vi "timeSeries.vi"(0 "Results Path":string="C:\\Users\\Hesham\\Desktop\\Analyse WT Data\\C1\\tmseries\\node1\\") -> (1 "Mean VRs":dbl[][](array[numeric]), 2 "GEM VRs":dbl[][](array[numeric]))   [LabVIEW 2018]
uses:
  <vilib>/Analysis/3filter.llb/Filter Passband Type.ctl
  <vilib>/Analysis/baseanly.llb/Mean (DBL).vi
  <vilib>/Utility/file.llb/Read Delimited Spreadsheet (string).vi
  <vilib>/Analysis/3filter.llb/Butterworth Filter (DBL).vi
  <vilib>/Analysis/NI_AALBase.lvlib
panel:
  out "Iteration":i32
  out "Input VR RMS":dbl[][](array[numeric])
  out "Input VR AVG":dbl[][](array[numeric])
  out "Processed Array - RMS":dbl[][](array[numeric])
  out "Processed Array - Means":dbl[][](array[numeric])
  out "Raw Array":sgl[][][](array[numeric])
  out "path":path
  out "Data":sgl[](graph)
  # "TO DO:\n- Add MF and AF to the probability calculation\n- Probes that have moved/removed"
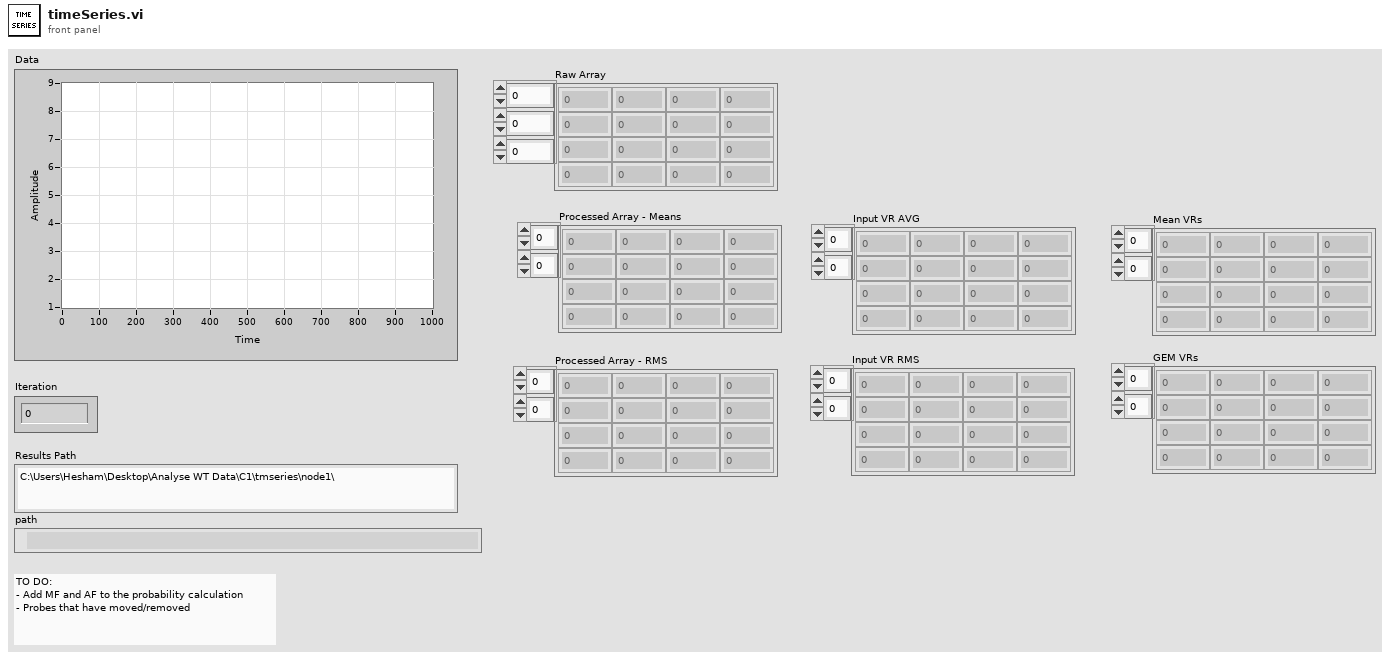
[diagram p1: front panel]
types:
  T1 = enum16{"big-endian, network order", "native, host order", "little-endian"}
  T2 = typedef "NI_AALBase.lvlib/Filter Passband Type.ctl" = enum32{"Lowpass", "Highpass", "Bandpass", "Bandstop"}
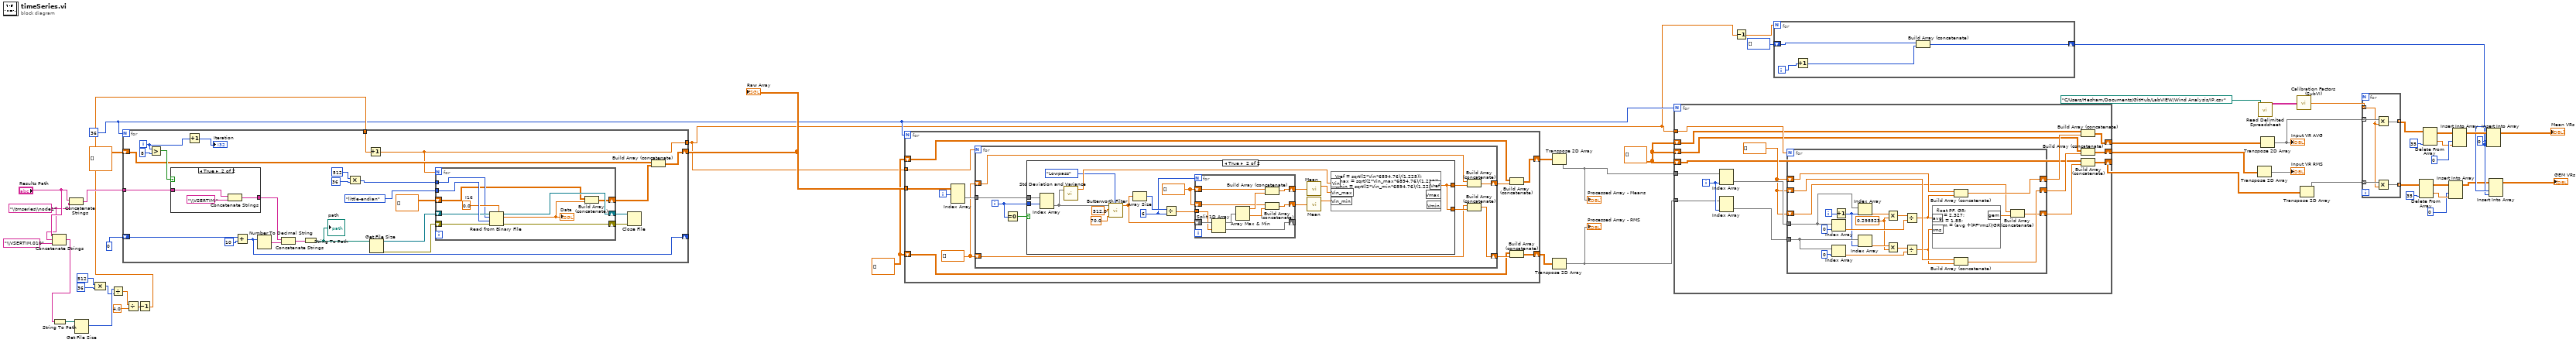
[diagram p0: block diagram]
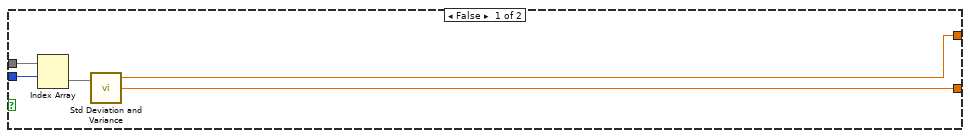
[diagram p2: hidden frame]
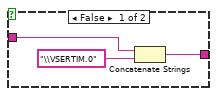
[diagram p3: hidden frame]
diagram:
  w4 = 0 ("disabled index (col)")
  w10 = 36
  w22 = "\\tmseries\\node1"
  w37 = dbl[][] []
  w42 = dbl[][] []
  n1 = Concatenate Strings("Results Path", w22, "\\VSERTIM.010" ("string")) -> (w20:string)
  n2 = String To Path(string=w20) -> (path=w19:path)
  n3 = Concatenate Strings("Results Path", w22) -> (w24:string)
  n4 = Get File Size(file=w19) -> (size (in bytes)=w18:i64)  [unwired: 1 in, 2 out]
  n5 = Compound Arithmetic op=MULTIPLY(512, 36 ("y")) -> (w15:i32)
  n6 = Divide(x=w18, y=w15) -> (x/y=w14:dbl)
  n7 = Divide(x=w14, y=4.0) -> (x/y=w12:dbl)
  n8 = Decrement(x=w12) -> (x-1=w11:dbl)
  n9 = for {
    N: w10 -> [_]
    shift-right: [w67] -> _
    shift-left: 0 -> [w68]
    tunnel: w24 -> [w64]
    shift-right: [w60] -> w50
    shift-left: sgl[][][] [] -> [w59]
    tunnel: [w57] -> w9
    tunnel: w11 -> [w53]
    i -> [w56]
    n10 = Greater?(x=w56, y=8) -> (0:w71:bool)
    n11 = case shown="True" w71 {
      tunnel: [w79 w82] -> w62
      tunnel: w64 -> [w81 w84]
      frame False {
        n12 = Concatenate Strings(w81, "\\VSERTIM.0") -> (w79:string)
      }
      frame True {
        n13 = Concatenate Strings(w84, "\\VSERTIM." ("string")) -> (w82:string)
      }
    }
    n14 = Increment(x=w56) -> (x+1=→"Iteration":i32)
    n15 = Add(x=w68, y=10) -> (x+y=w67:i32)
    n16 = Number To Decimal String(number=w67) -> (decimal integer string=w63:string)  [unwired: 1 in]
    n17 = Concatenate Strings(w62, w63) -> (w66:string)
    n18 = String To Path(string=w66) -> (path=w65:path)
    "path" <- w65
    n19 = Compound Arithmetic op=MULTIPLY(512, 36 ("y")) -> (w54:i32)
    n20 = Increment(x=w53) -> (x+1=w57:dbl)
    n21 = Get File Size(file=w65) -> (refnum out=w76:refnum<file>, 0:w77:errorcluster)  [unwired: 1 in, 1 out]
    n22 = for {
      N: w57 -> [_]
      tunnel: T1."little-endian" ("Byte Order") -> [w94]
      shift-right: [w89] -> w74
      shift-left: w77 -> [w93]
      shift-right: [w90] -> w75
      shift-left: w76 -> [w92]
      tunnel: w54 -> [w88]
      shift-right: [w86] -> w58
      shift-left: sgl[][] [] -> [w85]
      w91 = sgl 0.0  # I16
      n23 = Read from Binary File(5:w91, 8:w93, 9:w94, 10:w88, 11:w92) -> (0:w89:errorcluster, 2:w87:sgl[], 3:w90:refnum<file>)  [unwired: 1 in, 1 out]
      "Data" <- w87
      n24 = Build Array (concatenate)(w85, w87) -> (w86:sgl[][])
    }
    n25 = Close File(refnum=w75, error in=w74) -> ()  [unwired: 2 out]
    n26 = Build Array (concatenate)(w59, w58) -> (w60:sgl[][][])
  }
  "Raw Array" <- w50
  n27 = for {
    N: w10 -> [_]
    tunnel: w50 -> [w105]
    tunnel: w9 -> [w103]
    shift-right: [w101] -> w49
    shift-left: w42 -> [w100]
    shift-right: [w98] -> w48
    shift-left: w42 -> [w97]
    i -> [w104]
    w95 = dbl[] []
    n28 = Index Array(array=w105, index (dim 0)=w104) -> (element=w96:sgl[][])  [unwired: 2 in]
    n29 = for {
      N: w103 -> [_]
      tunnel: w96 -> [w111]
      shift-right: [w114] -> w102
      shift-left: w95 -> [w107]
      shift-right: [w113] -> w99
      shift-left: w95 -> [w106]
      i -> [w110]
      n30 = Equal To 0?(x=w110) -> (x = 0?=w112:bool)
      n31 = case shown="True" w112 {
        tunnel: w110 -> [w116 w136]
        tunnel: w111 -> [w119 w135]
        tunnel: [w117 w124] -> w108
        tunnel: [w118 w124] -> w109
        frame False {
          n32 = Index Array(array=w119, index (row)=w116) -> (element=w115:sgl[])  [unwired: 1 in]
          n33 = call <vilib>:"Std Deviation and Variance.vi"("X"=w115) -> ("mean"=w117:dbl, "standard deviation"=w118:dbl)  [unwired: 1 in, 1 out]
        }
        frame True {
          w127 = dbl[] []
          w122 = 6
          n34 = Index Array(array=w135, index (row)=w136) -> (element=w128:sgl[])  [unwired: 1 in]
          n35 = call <vilib>:"Std Deviation and Variance.vi"("X"=w128) -> ("mean"=w134:dbl)  [unwired: 1 in, 2 out]
          n36 = call-poly <vilib>:"Butterworth Filter.vi"("filter type"=Filter_Passband_Type."Lowpass", "low cutoff freq: fl"=70.0, "sampling freq: fs"=512.0, "X"=w128) -> ("Filtered X"=w121:dbl[])  [unwired: 4 in, 1 out]
          n37 = Array Size(array=w121) -> (size(s)=w123:i32)
          n38 = Divide(x=w123, y=w122) -> (x/y=w120:dbl)
          n39 = for {
            N: w122 -> [_]
            shift-right: [w145] -> _
            shift-left: w121 -> [w146]
            shift-right: [w144] -> w130
            shift-left: w127 -> [w141]
            shift-right: [w142] -> w129
            shift-left: w127 -> [w138]
            tunnel: w120 -> [w137]
            n40 = Split 1D Array(array=w146, index=w137) -> (first subarray=w143:dbl[], second subarray=w145:dbl[])
            n41 = Array Max & Min(array=w143) -> (max value=w140:dbl, min value=w139:dbl)  [unwired: 2 out]
            n42 = Build Array (concatenate)(w141, w140) -> (w144:dbl[])
            n43 = Build Array (concatenate)(w138, w139) -> (w142:dbl[])
          }
          n44 = call-poly <vilib>:"Mean.vi"("X"=w130) -> ("mean"=w126:dbl)  [unwired: 1 out]
          n45 = call-poly <vilib>:"Mean.vi"("X"=w129) -> ("mean"=w125:dbl)  [unwired: 1 out]
          n46 = formula code="Vref = sqrt((2*Vin*6894.76)/(1.225));\nVmax = sqrt((2*Vin_max*6894.76)/(1.225));\nVmin = sqrt((2*Vin_min*6894.76)/(1.225));"("Vin"=w134, "Vin_max"=w126, "Vin_min"=w125) -> ("Vref"=w124:dbl)  [unwired: 2 out]
        }
      }
      n47 = Build Array (concatenate)(w107, w108) -> (w114:dbl[])
      n48 = Build Array (concatenate)(w106, w109) -> (w113:dbl[])
    }
    n49 = Build Array (concatenate)(w100, w102) -> (w101:dbl[][])
    n50 = Build Array (concatenate)(w97, w99) -> (w98:dbl[][])
  }
  n51 = Transpose 2D Array(2D array=w49) -> (transposed array=w47:dbl[][])
  "Processed Array - Means" <- w47
  n52 = Transpose 2D Array(2D array=w48) -> (transposed array=w43:dbl[][])
  "Processed Array - RMS" <- w43
  n53 = for {
    N: w10 -> [_]
    tunnel: w47 -> [w157]
    tunnel: w9 -> [w161]
    shift-right: [w155] -> w46
    shift-left: w37 -> [w159]
    shift-right: [w153] -> w45
    shift-left: w37 -> [w152]
    tunnel: w43 -> [w151]
    shift-right: [w148] -> w36
    shift-left: w37 -> [w147]
    i -> [w158]
    w150 = dbl[] []
    n54 = Index Array(array=w157, index (col)=w158) -> (element=w162:dbl[])  [unwired: 1 in]
    n55 = Index Array(array=w151, index (col)=w158) -> (element=w156:dbl[])  [unwired: 1 in]
    n56 = for {
      N: w161 -> [_]
      tunnel: w162 -> [w176]
      shift-right: [w181] -> w160
      shift-left: w150 -> [w180]
      tunnel: w156 -> [w175]
      shift-right: [w170] -> w154
      shift-left: w150 -> [w169]
      shift-right: [w164] -> w149
      shift-left: w150 -> [w163]
      i -> [w183]
      w168 = 0.298523 ("y")
      n57 = Index Array(array=w176, index=0 ("index (row)")) -> (element=w182:dbl)
      n58 = Index Array(array=w175, index=0 ("index (row)")) -> (element=w172:dbl)
      n59 = Increment(x=w183) -> (x+1=w174:i32)
      n60 = Index Array(array=w176, index=w174) -> (element=w179:dbl)
      n61 = Index Array(array=w175, index=w174) -> (element=w171:dbl)
      n62 = Multiply(x=w179, y=w168) -> (x*y=w178:dbl)
      n63 = Multiply(x=w171, y=w168) -> (x*y=w173:dbl)
      n64 = Divide(x=w178, y=w182) -> (x/y=w167:dbl)
      n65 = Divide(x=w173, y=w172) -> (x/y=w166:dbl)
      n66 = formula code="float PF, GR; \nPF = 2.327;\nGR = 1.85;\ngem = (avg +(PF*rms))/GR;"("avg"=w167, "rms"=w166) -> ("gem"=w165:dbl)
      n67 = Build Array (concatenate)(w180, w167) -> (w181:dbl[])
      n68 = Build Array (concatenate)(w169, w166) -> (w170:dbl[])
      n69 = Build Array (concatenate)(w163, w165) -> (w164:dbl[])
    }
    n70 = Build Array (concatenate)(w159, w160) -> (w155:dbl[][])
    n71 = Build Array (concatenate)(w152, w154) -> (w153:dbl[][])
    n72 = Build Array (concatenate)(w147, w149) -> (w148:dbl[][])
  }
  n73 = Decrement(x=w9) -> (x-1=w8:dbl)
  n74 = for {
    N: w8 -> [_]
    shift-right: [w188] -> w3
    shift-left: i32[] [] -> [w187]
    i -> [w186]
    n75 = Increment(x=w186) -> (x+1=w185:i32)
    n76 = Build Array (concatenate)(w187, w185) -> (w188:i32[])
  }
  n77 = Transpose 2D Array(2D array=w45) -> (transposed array=→"Input VR RMS":dbl[][])
  n78 = call-poly <vilib>:"Read Delimited Spreadsheet.vi"("file path (dialog if empty)"=path "C:/Users/Hesham/Documents/GitHub/LabVIEW/Wind Analysis/IP.csv") -> ("all rows"=w41:string[][])  [unwired: 9 in, 5 out]
  n79 = Transpose 2D Array(2D array=w46) -> (transposed array=w39:dbl[][])
  "Input VR AVG" <- w39
  n80 = call "Calibration Factors (SubVI).vi"("IP List"=w41) -> ("Calibration Factors"=w38:dbl[])
  n81 = Transpose 2D Array(2D array=w36) -> (transposed array=w35:dbl[][])
  n82 = for {
    tunnel: w39 -> [w193] mode=indexing
    tunnel: w38 -> [w190] mode=indexing
    tunnel: [w192] -> w33 mode=indexing
    tunnel: w35 -> [w191] mode=indexing
    tunnel: [w189] -> w25 mode=indexing
    n83 = Multiply(x=w193, y=w190) -> (x*y=w192:dbl[])
    n84 = Multiply(x=w191, y=w190) -> (x*y=w189:dbl[])
  }
  n85 = Delete From Array(array=w25, index (col)=35 ("disabled index (col)")) -> (deleted portion=w29:dbl[], array with subset deleted=w27:dbl[][])  [unwired: 2 in]
  n86 = Delete From Array(array=w33, index (col)=35 ("disabled index (col)")) -> (deleted portion=w30:dbl[], array with subset deleted=w32:dbl[][])  [unwired: 2 in]
  n87 = Insert Into Array(array=w27, index (col)=0 ("disabled index (col)"), new element=w29) -> (w2:dbl[][])  [unwired: 1 in]
  n88 = Insert Into Array(array=w32, index (col)=0 ("disabled index (col)"), new element=w30) -> (w6:dbl[][])  [unwired: 1 in]
  n89 = Insert Into Array(array=w6, index (col)=w4, new element=w3) -> (→"Mean VRs":dbl[][])  [unwired: 1 in]
  n90 = Insert Into Array(array=w2, index (col)=w4, new element=w3) -> (→"GEM VRs":dbl[][])  [unwired: 1 in]
